vi "CRYGet New Cal Curves.vi"(6 "Hardware Channel infor Array In":T1[](array[typedef]) {"Coupling" items=["Default"=-1, "RSE"=10083, "NRSE"=10078, "Differential"=10106, "Pseudodifferential"=12529]; "term config" items=["Default"=-1, "RSE"=10083, "NRSE"=10078, "Differential"=10106, "Pseudodifferential"=12529]; "Anti-aliasing Factor (%fs)" format="%.2f"}, 8 "In/Out?":bool, 9 "Calibration 2D Array In":T2[](array[typedef]) {"Sens Curve"."Z data" items=["dB", "Lin"]; "Sens Curve"."X data" items=["dB", "Lin"]; "Sens Curve"."Y data" items=["dB", "Lin"]; "Sens Curve"."Z dB ref" format="%.1f"; "Sens Curve"."Z axis" items=["Log", "Lin"]; "Sens Curve"."X dB ref" format="%.1f"; "Sens Curve"."X axis" items=["Log", "Lin"]; "Sens Curve"."Y axis" items=["Log", "Lin"]; "Sens Curve"."Y dB ref" format="%.1f"; "Sens Curve"."Curve"."z" format="%.2f"; "Sens Curve"."Curve"."y" format="%.2f"; "Sens Curve"."Curve"."x" format="%.2f"; "EQ Curve"."Z data" items=["dB", "Lin"]; "EQ Curve"."X data" items=["dB", "Lin"]; "EQ Curve"."Y data" items=["dB", "Lin"]; "EQ Curve"."Z dB ref" format="%.1f"; "EQ Curve"."Z axis" items=["Log", "Lin"]; "EQ Curve"."X dB ref" format="%.1f"; "EQ Curve"."X axis" items=["Log", "Lin"]; "EQ Curve"."Y axis" items=["Log", "Lin"]; "EQ Curve"."Y dB ref" format="%.1f"; "EQ Curve"."Curve"."z" format="%.2f"; "EQ Curve"."Curve"."y" format="%.2f"; "EQ Curve"."Curve"."x" format="%.2f"; "Corr Curve"."Z data" items=["dB", "Lin"]; "Corr Curve"."X data" items=["dB", "Lin"]; "Corr Curve"."Y data" items=["dB", "Lin"]; "Corr Curve"."Z dB ref" format="%.1f"; "Corr Curve"."Z axis" items=["Log", "Lin"]; "Corr Curve"."X dB ref" format="%.1f"; "Corr Curve"."X axis" items=["Log", "Lin"]; "Corr Curve"."Y axis" items=["Log", "Lin"]; "Corr Curve"."Y dB ref" format="%.1f"; "Corr Curve"."Curve"."z" format="%.2f"; "Corr Curve"."Curve"."y" format="%.2f"; "Corr Curve"."Curve"."x" format="%.2f"; "Calibration"."EQ Step size" items=["R10", "R20", "R40", "R80", "User"]; "Calibration"."Corr Step size" items=["R10", "R20", "R40", "R80", "User"]}, 11 "Name In":string[][](array[string])) -> (0 "Detail Information Out":string[][](array[string]), 3 "Calibration 2D Array Out":T2[](array[typedef]) {"Sens Curve"."Z data" items=["dB", "Lin"]; "Sens Curve"."X data" items=["dB", "Lin"]; "Sens Curve"."Y data" items=["dB", "Lin"]; "Sens Curve"."Z dB ref" format="%.1f"; "Sens Curve"."Z axis" items=["Log", "Lin"]; "Sens Curve"."X dB ref" format="%.1f"; "Sens Curve"."X axis" items=["Log", "Lin"]; "Sens Curve"."Y axis" items=["Log", "Lin"]; "Sens Curve"."Y dB ref" format="%.1f"; "Sens Curve"."Curve"."z" format="%.2f"; "Sens Curve"."Curve"."y" format="%.2f"; "Sens Curve"."Curve"."x" format="%.2f"; "EQ Curve"."Z data" items=["dB", "Lin"]; "EQ Curve"."X data" items=["dB", "Lin"]; "EQ Curve"."Y data" items=["dB", "Lin"]; "EQ Curve"."Z dB ref" format="%.1f"; "EQ Curve"."Z axis" items=["Log", "Lin"]; "EQ Curve"."X dB ref" format="%.1f"; "EQ Curve"."X axis" items=["Log", "Lin"]; "EQ Curve"."Y axis" items=["Log", "Lin"]; "EQ Curve"."Y dB ref" format="%.1f"; "EQ Curve"."Curve"."z" format="%.2f"; "EQ Curve"."Curve"."y" format="%.2f"; "EQ Curve"."Curve"."x" format="%.2f"; "Corr Curve"."Z data" items=["dB", "Lin"]; "Corr Curve"."X data" items=["dB", "Lin"]; "Corr Curve"."Y data" items=["dB", "Lin"]; "Corr Curve"."Z dB ref" format="%.1f"; "Corr Curve"."Z axis" items=["Log", "Lin"]; "Corr Curve"."X dB ref" format="%.1f"; "Corr Curve"."X axis" items=["Log", "Lin"]; "Corr Curve"."Y axis" items=["Log", "Lin"]; "Corr Curve"."Y dB ref" format="%.1f"; "Corr Curve"."Curve"."z" format="%.2f"; "Corr Curve"."Curve"."y" format="%.2f"; "Corr Curve"."Curve"."x" format="%.2f"; "Calibration"."EQ Step size" items=["R10", "R20", "R40", "R80", "User"]; "Calibration"."Corr Step size" items=["R10", "R20", "R40", "R80", "User"]})   [LabVIEW 2013]
uses:
  Typedef Control/CRYCalibration 2DCluster.ctl
  Typedef Control/CRYCalibration Cluster.ctl
  Typedef Control/CRYData Cluster.ctl
  Typedef Control/CRYHardware Channel Info.ctl
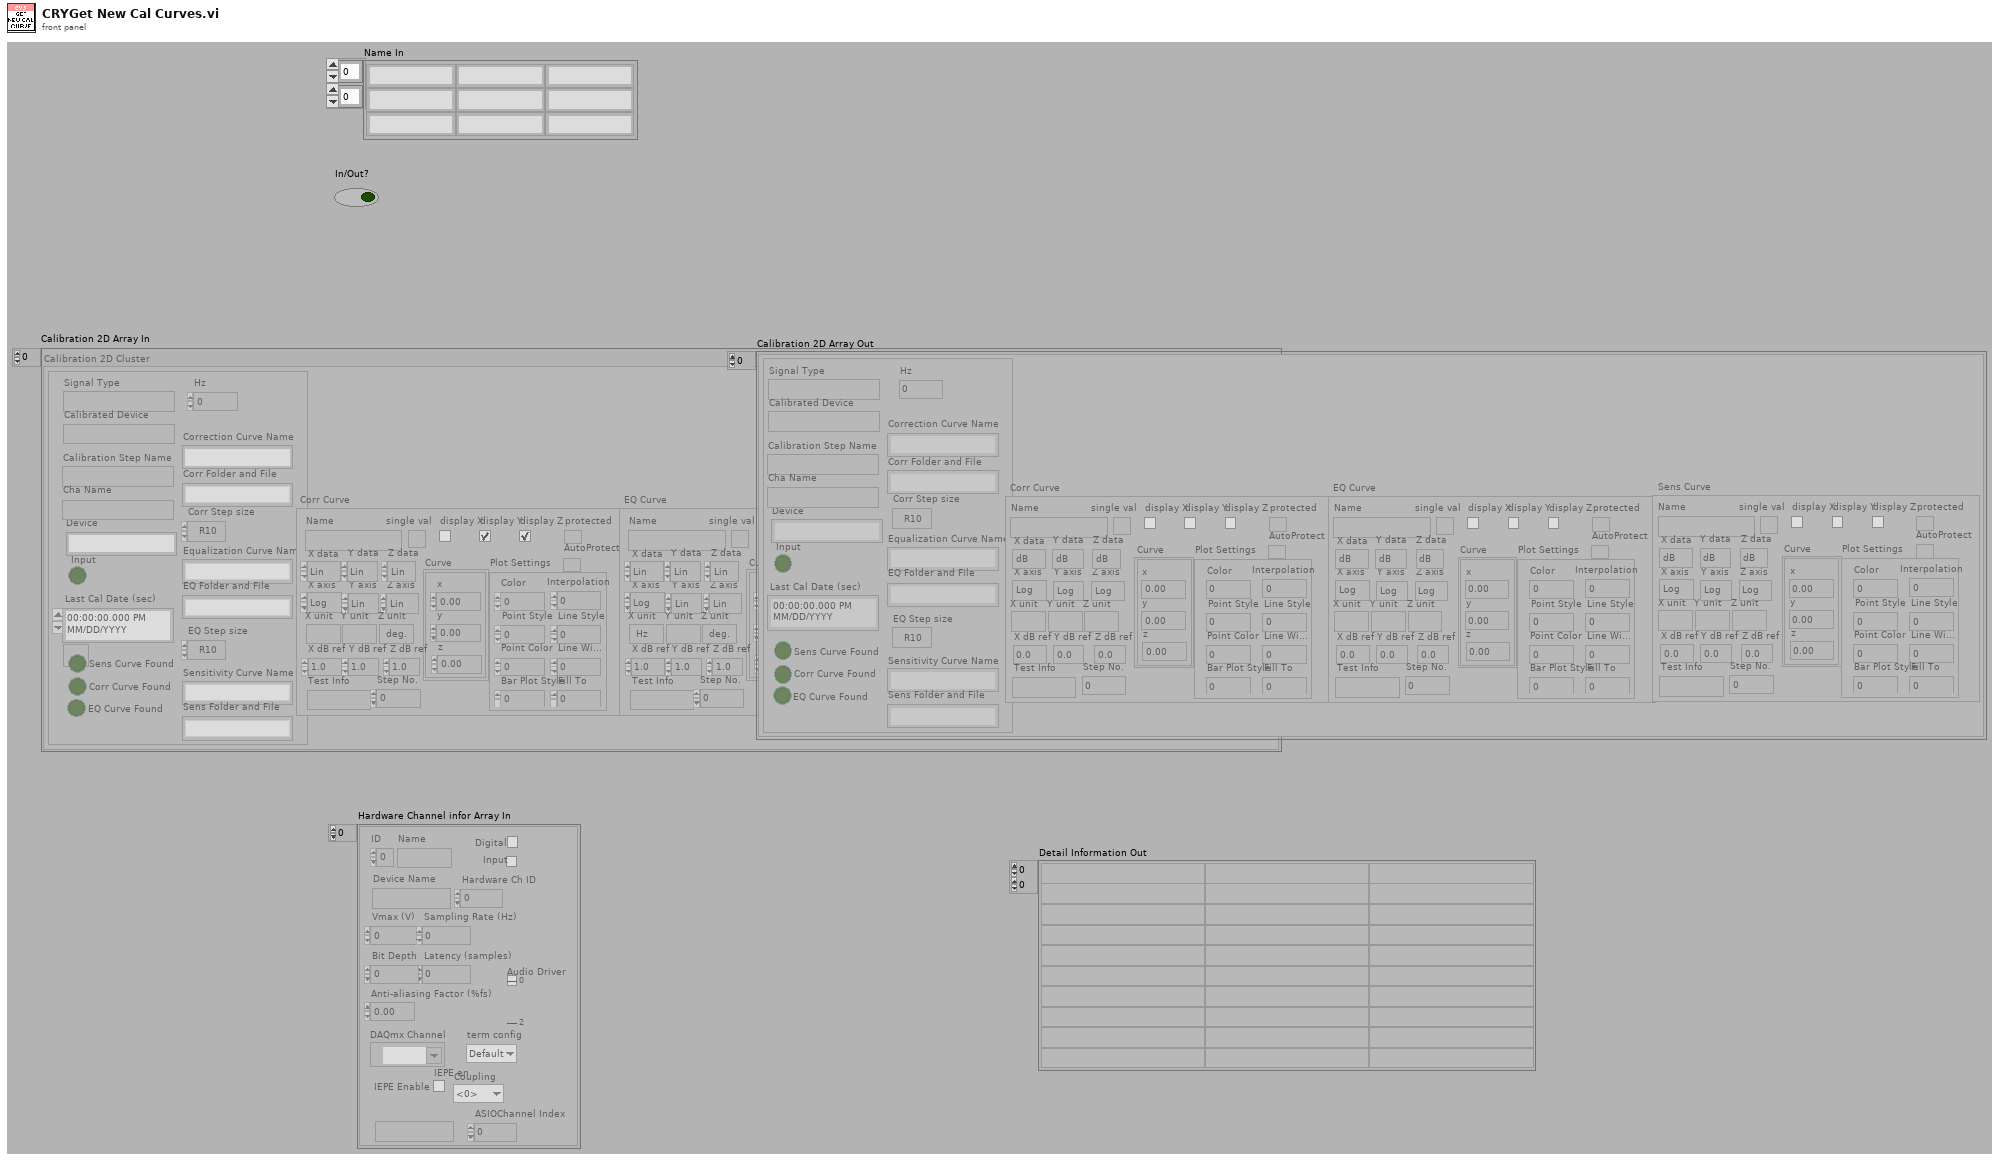
[diagram p1: front panel]
types:
  T1 = typedef "CRYHardware Channel Info.ctl" = cluster{"ID":i32, "Name":string, "Digital":bool, "Input":bool, "Device Name":string, "Hardware Ch ID":u8, "Vmax (V)":dbl, "Latency (samples)":dbl, "Sampling Rate (Hz)":u32, "Bit Depth":u32, "Anti-aliasing Factor (%fs)":sgl, "DAQmx Channel":tag, "term config":i32, "Coupling":i32, "IEPE en":bool, "ASIOChannel Name":string, "Audio Driver":u16, "ASIOChannel Index":u8}
  T2 = typedef "CRYCalibration 2DCluster.ctl" = cluster{"Calibration":T3, "Corr Curve":T4, "EQ Curve":T4, "Sens Curve":T4}
  T3 = typedef "CRYCalibration Cluster.ctl" = cluster{"Calibration Step Name":string, "Device":string, "Correction Curve Name":string, "Equalization Curve Name":string, "Sensitivity Curve Name":string, "Corr Folder and File":string, "EQ Folder and File":string, "Sens Folder and File":string, "Corr Step size":u16, "EQ Step size":u16, "Input":bool, "Last Cal Date (sec)":timestamp, "Cha Name":string, "Corr Curve Found":bool, "EQ Curve Found":bool, "Sens Curve Found":bool, "Signal Type":string, "Calibrated Device":string, "Hz":u32}
  T4 = typedef "CRYData Cluster.ctl" = cluster{"Name":string, "Curve":cluster{"x":dbl, "y":dbl, "z":dbl}[], "X data":u16, "Y data":u16, "Z data":u16, "X axis":u16, "Y axis":u16, "Z axis":u16, "X unit":string, "Y unit":string, "Z unit":string, "X dB ref":dbl, "Y dB ref":dbl, "Z dB ref":dbl, "single val":bool, "protected":bool, "display X":bool, "display Y":bool, "display Z":bool, "Test Info":string, "Step No.":i32, "Plot Settings":cluster{"Color":u32, "Interpolation":u8, "Point Style":u8, "Line Style":u8, "Point Color":u32, "Line Width":u8, "Bar Plot Style":u8, "Fill To":i16}, "AutoProtect":bool}
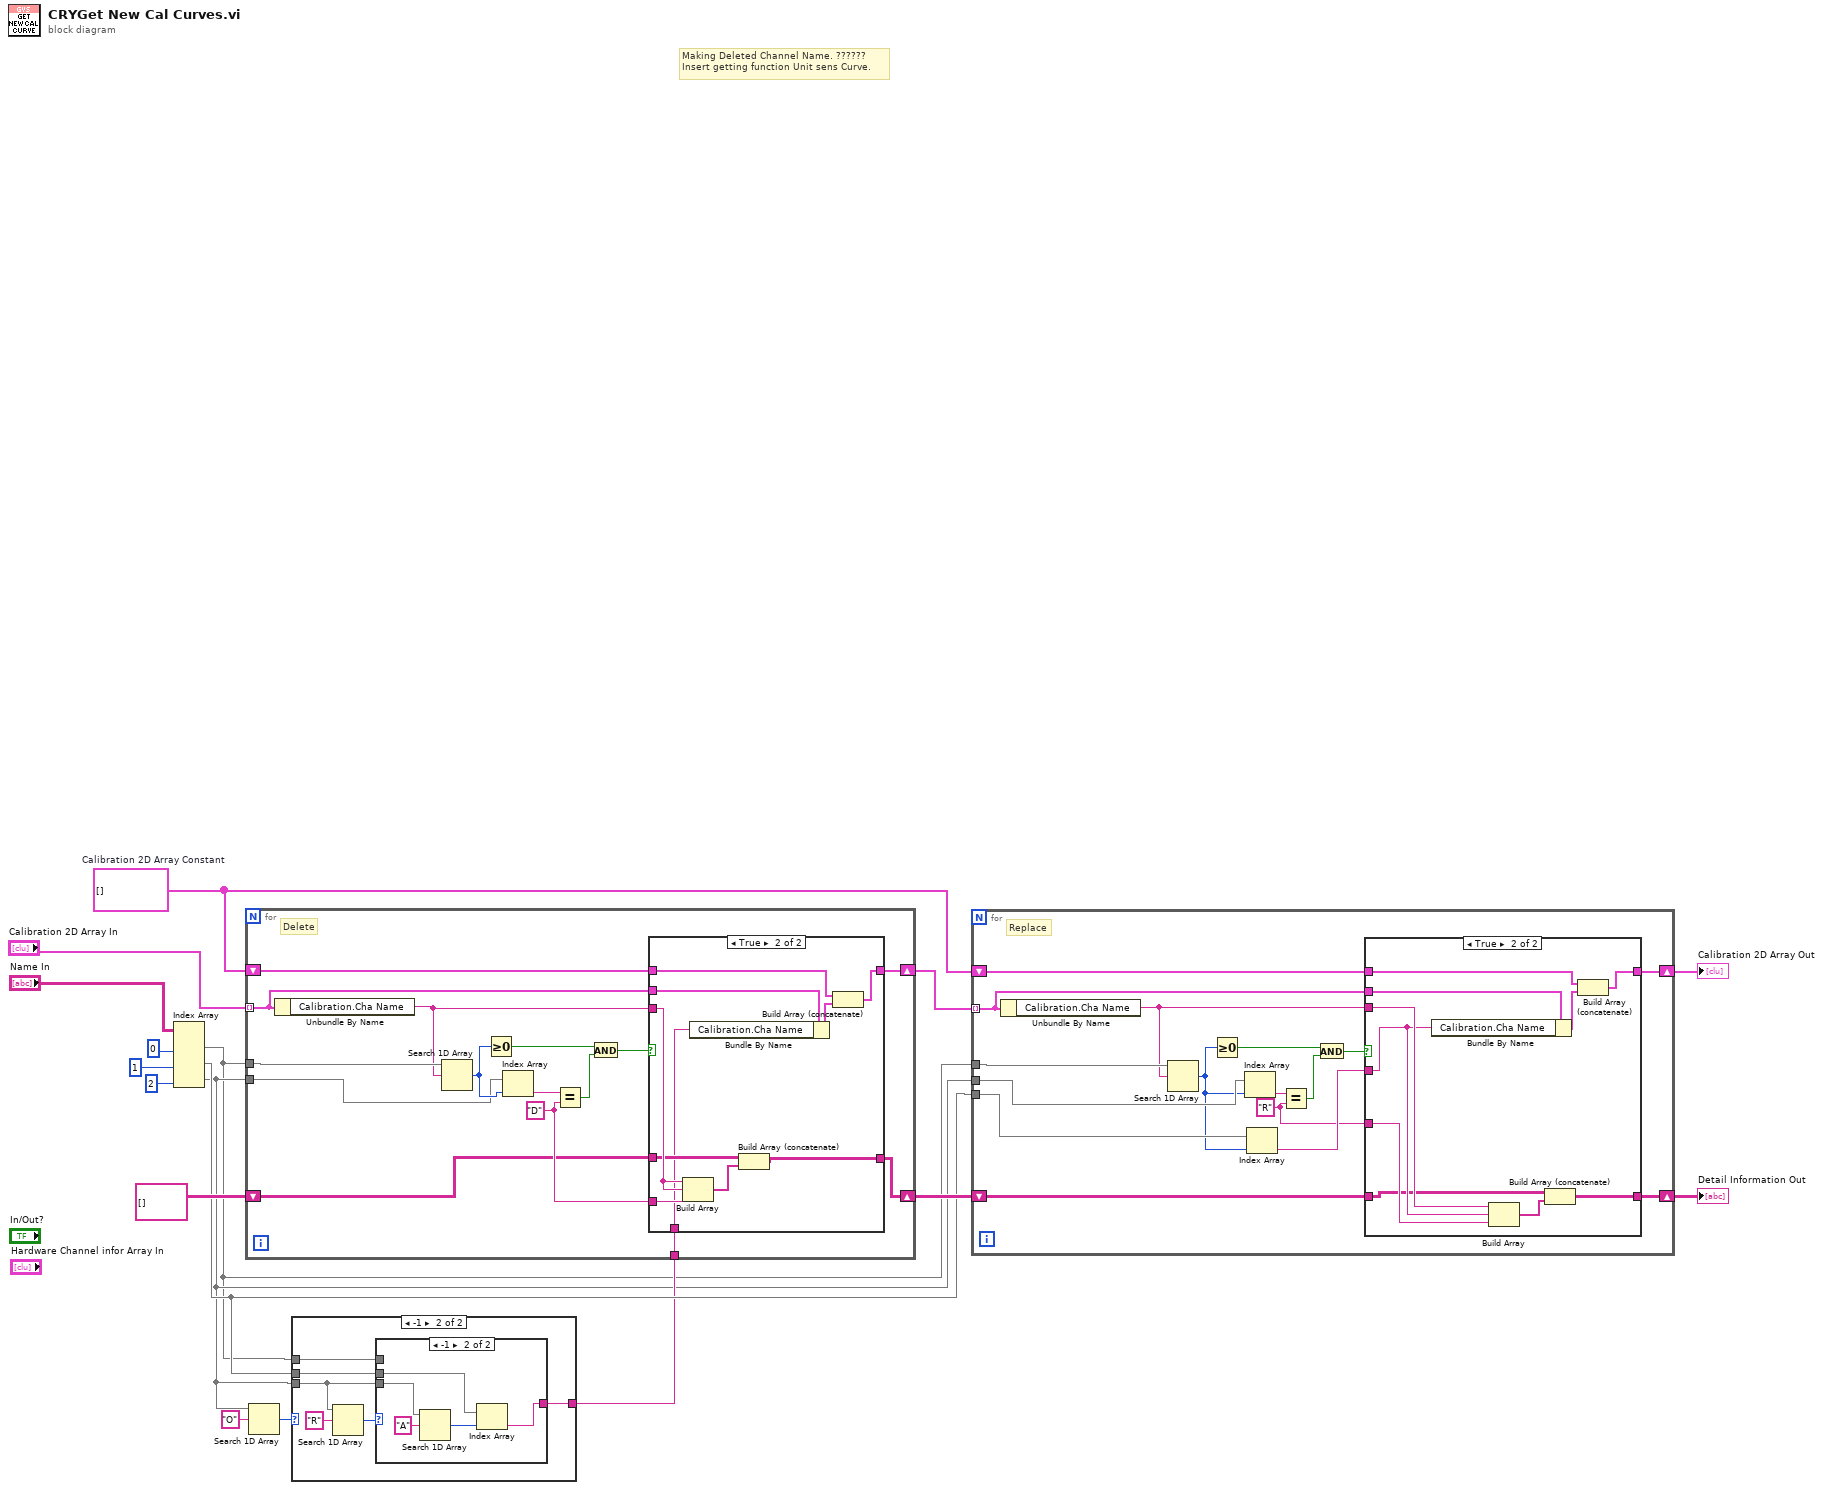
[diagram p0: block diagram]
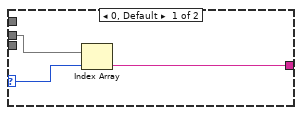
[diagram p2: hidden frame]
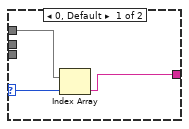
[diagram p3: hidden frame]
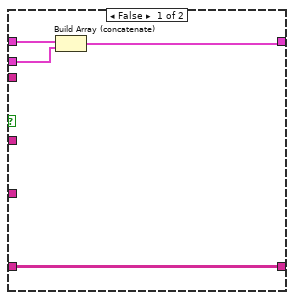
[diagram p4: hidden frame]
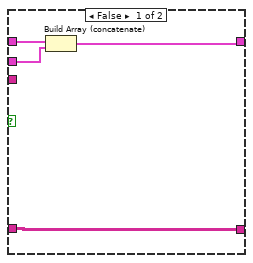
[diagram p5: hidden frame]
diagram:
  w11 = T2[] []  # Calibration 2D Array Constant
  # "Making Deleted Channel Name. ??????\nInsert getting function Unit sens Curve."
  n1 = Index Array(array="Name In", index (col) #1=0 ("index"), index (col) #2=1 ("index"), index (col) #3=2 ("index")) -> (element #1=w1:string[], element #2=w4:string[], element #3=w2:string[])  [unwired: 3 in]
  n2 = Search 1D Array(1D array=w2, element="O") -> (index of element=w5:i32)  [unwired: 1 in]
  n3 = case shown="-1" w5 {
    selector: w5 -> [w20 _]
    tunnel: w4 -> [w19 w23]
    tunnel: [w18 w22] -> w3
    tunnel: w2 -> [_ w24]
    tunnel: w1 -> [_ w21]
    frame 0, Default {
      n4 = Index Array(array=w19, index=w20) -> (element=w18:string)
    }
    frame -1 {
      n5 = Search 1D Array(1D array=w24, element="R") -> (index of element=w25:i32)  [unwired: 1 in]
      n6 = case shown="-1" w25 {
        selector: w25 -> [w29 _]
        tunnel: w24 -> [_ w33]
        tunnel: w23 -> [_ w31]
        tunnel: [w28 w30] -> w22
        tunnel: w21 -> [w27 _]
        frame 0, Default {
          n7 = Index Array(array=w27, index=w29) -> (element=w28:string)
        }
        frame -1 {
          n8 = Search 1D Array(1D array=w33, element="A") -> (index of element=w32:i32)  [unwired: 1 in]
          n9 = Index Array(array=w31, index=w32) -> (element=w30:string)
        }
      }
    }
  }
  n10 = for {
    tunnel: "Calibration 2D Array In" -> [w47] mode=indexing
    shift-right: [w48] -> w12
    shift-left: w11 -> [w49]
    tunnel: w1 -> [w46]
    tunnel: w2 -> [w44]
    shift-right: [w36] -> w8
    shift-left: string[][] [] ("Array") -> [w37]
    tunnel: w3 -> [w35]
    w39 = "D" ("y")
    # "Delete"
    n11 = Unbundle By Name(w47) -> ("Calibration.Cha Name"=w38:string)
    n12 = Search 1D Array(1D array=w46, element=w38) -> (index of element=w45:i32)  [unwired: 1 in]
    n13 = Greater Or Equal To 0?(x=w45) -> (x >= 0?=w41:bool)
    n14 = Index Array(array=w44, index=w45) -> (element=w43:string)
    n15 = Equal?(x=w43, y=w39) -> (x = y?=w42:bool)
    n16 = And(x=w41, y=w42) -> (x .and. y?=w40:bool)
    n17 = case shown="True" w40 {
      tunnel: w49 -> [w53 w58]
      tunnel: [w52 w57] -> w48
      tunnel: w47 -> [w51 w56]
      tunnel: w39 -> [_ w63]
      tunnel: w38 -> [_ w62]
      tunnel: w37 -> [w50 w61]
      tunnel: [w50 w59] -> w36
      tunnel: w35 -> [_ w54]
      frame False {
        n18 = Build Array (concatenate)(w53, w51) -> (w52:T2[])
      }
      frame True {
        n19 = Build Array(w62, w62, w63) -> (w60:string[])
        n20 = Bundle By Name(cluster=w56, "Calibration.Cha Name"=w54) -> (w55:T2)
        n21 = Build Array (concatenate)(w61, w60) -> (w59:string[][])
        n22 = Build Array (concatenate)(w58, w55) -> (w57:T2[])
      }
    }
  }
  n23 = for {
    tunnel: w12 -> [w69] mode=indexing
    shift-right: [w78] -> w10
    shift-left: w11 -> [w79]
    tunnel: w1 -> [w77]
    tunnel: w2 -> [w76]
    tunnel: w4 -> [w71]
    shift-right: [w64] -> w7
    shift-left: w8 -> [w67]
    w66 = "R" ("y")
    # "Replace"
    n24 = Unbundle By Name(w69) -> ("Calibration.Cha Name"=w65:string)
    n25 = Search 1D Array(1D array=w77, element=w65) -> (index of element=w70:i32)  [unwired: 1 in]
    n26 = Greater Or Equal To 0?(x=w70) -> (x >= 0?=w73:bool)
    n27 = Index Array(array=w76, index=w70) -> (element=w75:string)
    n28 = Index Array(array=w71, index=w70) -> (element=w68:string)
    n29 = Equal?(x=w75, y=w66) -> (x = y?=w74:bool)
    n30 = And(x=w73, y=w74) -> (x .and. y?=w72:bool)
    n31 = case shown="True" w72 {
      tunnel: w79 -> [w83 w91]
      tunnel: [w82 w90] -> w78
      tunnel: w69 -> [w81 w93]
      tunnel: w68 -> [_ w87]
      tunnel: w67 -> [w80 w86]
      tunnel: w66 -> [_ w89]
      tunnel: w65 -> [_ w88]
      tunnel: [w80 w84] -> w64
      frame False {
        n32 = Build Array (concatenate)(w83, w81) -> (w82:T2[])
      }
      frame True {
        n33 = Bundle By Name(cluster=w93, "Calibration.Cha Name"=w87) -> (w92:T2)
        n34 = Build Array(w88, w87, w89) -> (w85:string[])
        n35 = Build Array (concatenate)(w86, w85) -> (w84:string[][])
        n36 = Build Array (concatenate)(w91, w92) -> (w90:T2[])
      }
    }
  }
  "Calibration 2D Array Out" <- w10
  "Detail Information Out" <- w7
